vi "check if tag select name exists.vi"(10 "name to locate":string, 11 "tag select module configuration in":refnum<class "tag select module configuration.lvclass">) -> (0 "tag select config":T1, 1 "index":i32, 2 "found?":bool, 3 "tag select module configuration out":refnum<class "tag select module configuration.lvclass">)   [LabVIEW 2013, in "tag select module configuration.lvclass"]
uses:
  tag select module configuration.lvclass
  tag select configuration.ctl
  <vilib>/NI/Tag Bus Module Framework/channel/TBM channel.lvclass
  <vilib>/NI/Tag Bus/tag/Data Type.ctl
  tag select module configuration.lvclass/tag select module configuration.ctl
  <vilib>/NI/Tag Bus/tag/tag descriptor.lvclass
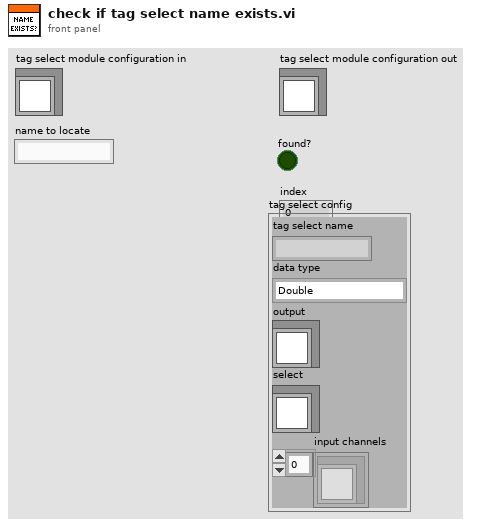
[diagram p1: front panel]
types:
  T1 = typedef "tag select module configuration.lvclass/tag select configuration.ctl" = cluster{"tag select name":string, "data type":T2, "output":refnum<class "TBM channel.lvclass">, "select":refnum<class "TBM channel.lvclass">, "input channels":refnum<class "TBM channel.lvclass">[]}
  T2 = typedef "tag bus.lvlib/tag descriptor.lvclass/Data Type.ctl" = enum16{"Double", "Single", "I64", "I32", "I16", "I8", "U64", "U32", "U16", "U8", "Boolean", "String", "Array of Double", "Array of Single", "Array of I64", "Array of I32", "Array of I16", "Array of I8", "Array of U64", "Array of U32", "Array of U16", "Array of U8", "Array of Boolean", "Array of String"}
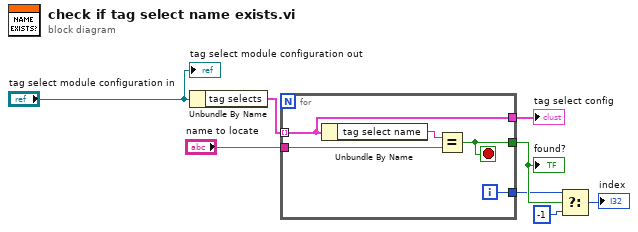
[diagram p0: block diagram]
diagram:
  n1 = Unbundle By Name("tag select module configuration in") -> ("tag selects"=w7:T1[])
  n2 = for {
    tunnel: w7 -> [w9] mode=indexing
    tunnel: "name to locate" -> [w12]
    tunnel: [w11] -> w5
    tunnel: [w10] -> w4
    tunnel: [w9] -> w1
    i -> [w10]
    stop <- w11 stop-if-true
    n3 = Unbundle By Name(w9) -> ("tag select name"=w13:string)
    n4 = Equal?(x=w13, y=w12) -> (x = y?=w11:bool)
  }
  "found?" <- w5
  "tag select config" <- w1
  n5 = Select(t=w4, s=w5, f=-1) -> (s? t:f=→"index":i32)
  "tag select module configuration out" <- "tag select module configuration in"
